vi "Single Project Checker.vi"(10 "VI and Library References":T1[](array[typedef])) -> (1 "Ref":T1, 2 "Target":string)   [LabVIEW 2020, in "_Shared.lvlib" / "Project Stuff.lvclass"]
uses:
  Project Stuff.lvclass
  <vilib>/Utility/EditLVProj/Library And VI References.ctl
  <vilib>/Utility/EditLVProj/Edit LVProj.lvlib
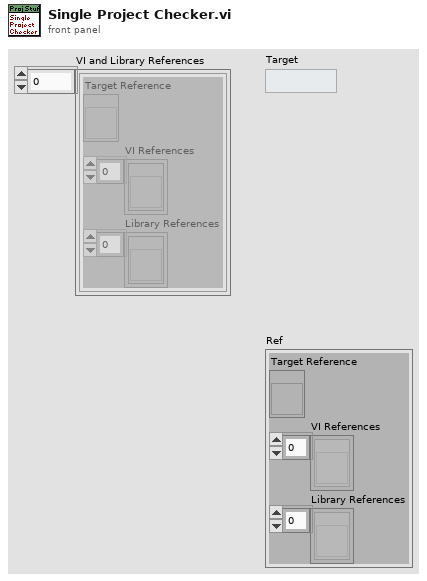
[diagram p1: front panel]
types:
  T1 = typedef "Edit LVProj.lvlib/Library And VI References.ctl" = cluster{"Target Reference":refnum<vi>, "VI References":refnum<vi>[], "Library References":refnum<vi>[]}
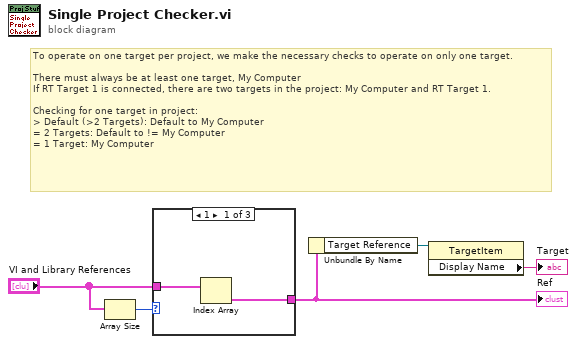
[diagram p0: block diagram]
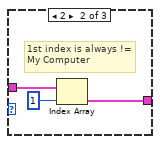
[diagram p2: hidden frame]
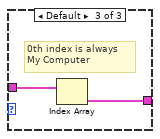
[diagram p3: hidden frame]
diagram:
  # "To operate on one target per project, we make the necessary checks to operate on only one target.\n\nThere must always be at least one target, My Computer\nIf RT Target 1 is connected, there are two targets in the project: My Computer and RT Target 1.\n\nChecking for one target in project:\n> Default (>2 Targets): Default to My Computer\n= 2 Targets: Default to != My Computer\n= 1 Target: My Computer"
  n1 = Array Size(array="VI and Library References") -> (size(s)=w3:i32)
  n2 = case shown="1" w3 {
    tunnel: "VI and Library References" -> [w7 w10 w12]
    tunnel: [w6 w8 w11] -> w1
    frame 1 {
      n3 = Index Array(array=w7) -> (element=w6:T1)  [unwired: 1 in]
    }
    frame 2 {
      # "1st index is always != My Computer"
      n4 = Index Array(array=w10, index=1) -> (element=w8:T1)
    }
    frame Default {
      # "0th index is always My Computer"
      n5 = Index Array(array=w12) -> (element=w11:T1)  [unwired: 1 in]
    }
  }
  "Ref" <- w1
  n6 = Unbundle By Name(w1) -> ("Target Reference"=w4:refnum<vi>)
  n7 = property class="TargetItem"(reference=w4) -> ("Display Name"=→"Target":string)  [unwired: 1 in, 2 out]
